vi "Set URI String.vi"(8 "error in (no error)":errorcluster, 10 "URI String":string, 11 "URI in":refnum<class "URI.lvclass">) -> (0 "error out":errorcluster, 3 "URI out":refnum<class "URI.lvclass">)   [LabVIEW 2020, in "URI.lvclass"]
uses:
  URI.lvclass
  URI.lvclass/URI.ctl
  <vilib>/regexp/Match Regular Expression.xnode
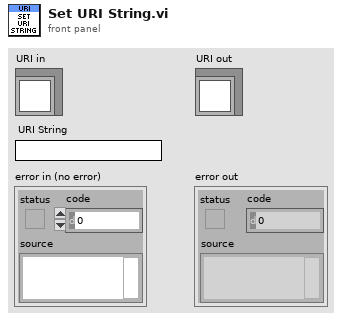
[diagram p1: front panel]
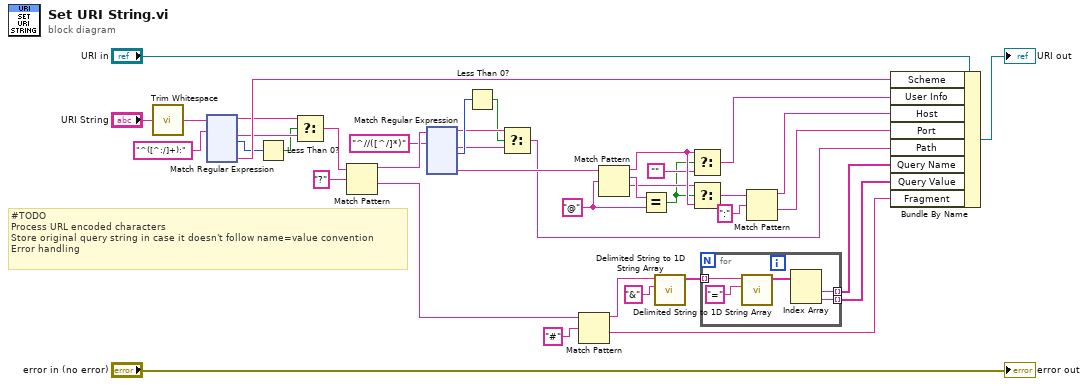
[diagram p0: block diagram]
diagram:
  w24 = "@" ("regular expression")
  # "#TODO\nProcess URL encoded characters\nStore original query string in case it doesn't follow name=value convention\nError handling"
  n1 = call <vilib>:"Trim Whitespace.vi"("string"="URI String") -> ("trimmed string"=w36:string)  [unwired: 1 in]
  n2 = xnode "Match Regular Expression"("input string"=w36, "regular expression"="^([^:/]+):") -> ("before match"=w33:string, "after match"=w32:string, "offset past match"=w31:i32, "submatch 1"=w34:string)  [unwired: 4 in, 2 out]
  n3 = Less Than 0?(x=w31) -> (x < 0?=w30:bool)
  n4 = Select(t=w33, s=w30, f=w32) -> (s? t:f=w29:string)
  n5 = Match Pattern(string=w29, regular expression="?") -> (before substring=w27:string, after substring=w12:string)  [unwired: 1 in, 2 out]
  n6 = xnode "Match Regular Expression"("input string"=w27, "regular expression"="^//([^/]*)") -> ("before match"=w4:string, "after match"=w3:string, "offset past match"=w5:i32, "submatch 1"=w25:string)  [unwired: 4 in, 2 out]
  n7 = Less Than 0?(x=w5) -> (x < 0?=w2:bool)
  n8 = Select(t=w4, s=w2, f=w3) -> (s? t:f=w1:string)
  n9 = Match Pattern(string=w12, regular expression="#") -> (before substring=w10:string, after substring=w11:string)  [unwired: 1 in, 2 out]
  n10 = Match Pattern(string=w25, regular expression=w24) -> (before substring=w22:string, match substring=w23:string, after substring=w20:string)  [unwired: 1 in, 1 out]
  n11 = Equal?(x=w23, y=w24) -> (x = y?=w19:bool)
  n12 = call <vilib>:"Delimited String to 1D String Array.vi"("delimiter"="&", "delimited string"=w10) -> ("string array"=w8:string[])  [unwired: 9 in]
  n13 = Select(t=w22, s=w19, f="") -> (s? t:f=w18:string)
  n14 = Select(t=w20, s=w19, f=w22) -> (s? t:f=w17:string)
  n15 = for {
    tunnel: w8 -> [w45] mode=indexing
    tunnel: [w42] -> w7 mode=indexing
    tunnel: [w41] -> w6 mode=indexing
    n16 = call <vilib>:"Delimited String to 1D String Array.vi"("delimiter"="=", "delimited string"=w45) -> ("string array"=w43:string[])  [unwired: 9 in]
    n17 = Index Array(array=w43) -> (element #1=w42:string, element #2=w41:string)  [unwired: 2 in]
  }
  n18 = Match Pattern(string=w17, regular expression=":") -> (before substring=w15:string, after substring=w14:string)  [unwired: 1 in, 2 out]
  n19 = Bundle By Name(cluster="URI in", "Scheme"=w34, "User Info"=w18, "Host"=w15, "Port"=w14, "Path"=w1, "Query Name"=w7, "Query Value"=w6, "Fragment"=w11) -> (→"URI out":refnum<class "URI.lvclass">)
  "error out" <- "error in (no error)"
